vi "FromMatlabParam.vi"(9 "IgnoreContainerName":bool, 10 "Matlab Param Data":T1[](array[typedef]), 11 "Type (or value to update)":variant) -> (3 "Value":variant)   [LabVIEW 2017]
uses:
  Types/MatlabDataBundle.ctl
  Types/MatlabDataType.ctl
  <vilib>/Utility/Data Type/NI_Data Type.lvlib
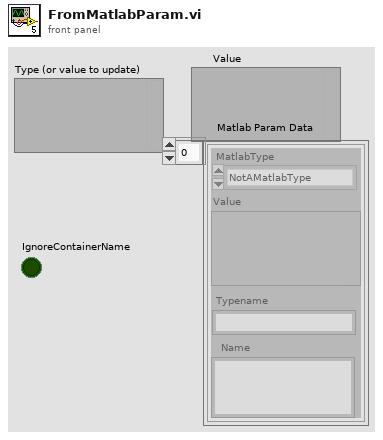
[diagram p1: front panel]
types:
  T1 = typedef "MatlabDataBundle.ctl" = cluster{"MatlabType":T2, "Value":variant, "Name":string, "Typename":string}
  T2 = typedef "MatlabDataType.ctl" = enum16{"NotAMatlabType", "Real", "Complex", "String", "Boolean"}
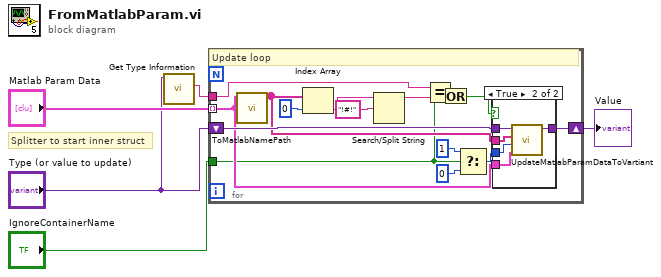
[diagram p0: block diagram]
diagram:
  # "Splitter to start inner struct"
  n1 = call <vilib>:"Get Type Information.vi"("Variant"="Type (or value to update)") -> ("Name"=w2:string)  [unwired: 6 in, 4 out]
  n2 = for {
    tunnel: "Matlab Param Data" -> [w18] mode=indexing
    shift-right: [w19] -> w4
    shift-left: "Type (or value to update)" -> [w20]
    tunnel: w2 -> [w6]
    tunnel: "IgnoreContainerName" -> [w13]
    # "Update loop"
    n3 = call "ToMatlabNamePath.vi"("MatlabDataBundle"=w18) -> ("NamePath"=w17:string[])  [unwired: 10 in]
    n4 = Index Array(array=w17, index=0) -> (element=w9:string)
    n5 = Search/Split String(string=w9, search string/char (-)="!#!") -> (substring before match=w7:string)  [unwired: 1 in, 2 out]
    n6 = Equal?(x=w6, y=w7) -> (x = y?=w15:bool)
    n7 = Or(x=w15, y=w13) -> (x .or. y?=w14:bool)
    n8 = Select(t=1, s=w13, f=0 ("index")) -> (s? t:f=w11:i32)
    n9 = case shown="True" w14 {
      tunnel: w20 -> [w21 w26]
      tunnel: [w21 w25] -> w19
      tunnel: w18 -> [_ w24]
      tunnel: w17 -> [_ w23]
      tunnel: w11 -> [_ w22]
      frame False {
      }
      frame True {
        n10 = call "UpdateMatlabParamDataToVartiant.vi"("MatlabDataBundle"=w24, "curNameIndex"=w22, "NamePath"=w23, "Type (or value to update)"=w26) -> ("Value"=w25:variant)  [unwired: 7 in]
      }
    }
  }
  "Value" <- w4
